vi "connection.list.vi"(8 "error in":errorcluster, 11 "Nominal Client in":refnum<class "Nominal Client.lvclass">) -> (0 "error out":errorcluster, 1 "Response":string, 2 "Nominal Connections":T1(array[cluster]), 3 "Nominal Client out":refnum<class "Nominal Client.lvclass">, 4 "Connections":T2(array[cluster]))   [LabVIEW 2024, in "nominal labview client.lvlib"]
uses:
  nominal labview client.lvlib
  <vilib>/Nominal/Nominal IO Client/Nominal Client/Nominal Client.lvclass
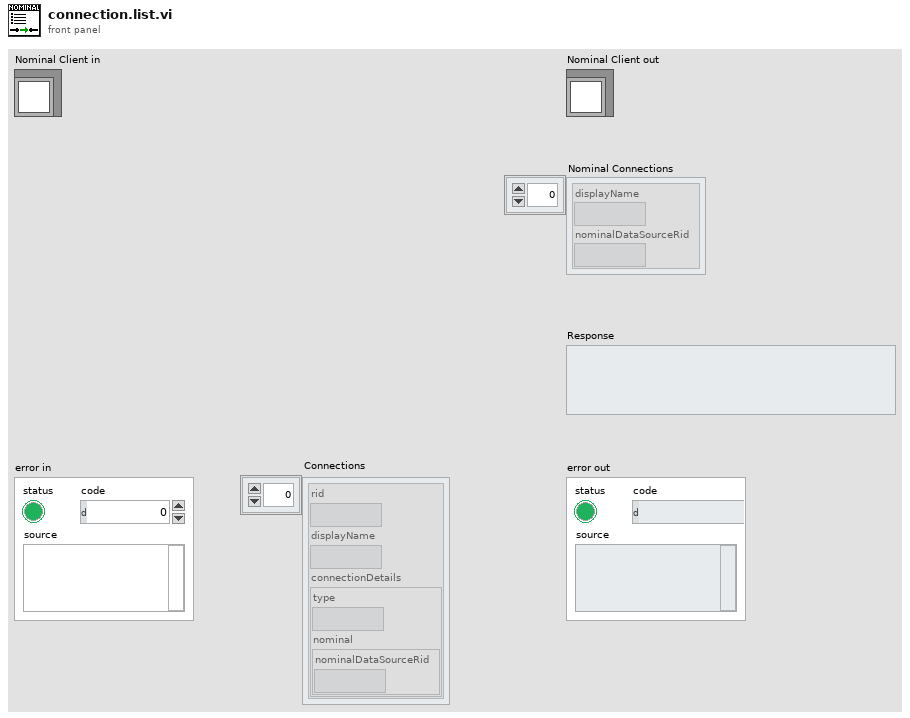
[diagram p1: front panel]
types:
  T1 = cluster{"displayName":string, "nominalDataSourceRid":string}[]
  T2 = cluster{"rid":string, "displayName":string, "connectionDetails":cluster{"type":string, "nominal":cluster{"nominalDataSourceRid":string}}}[]
  T3 = cluster{"displayName":string, "nominalDataSourceRid":string}
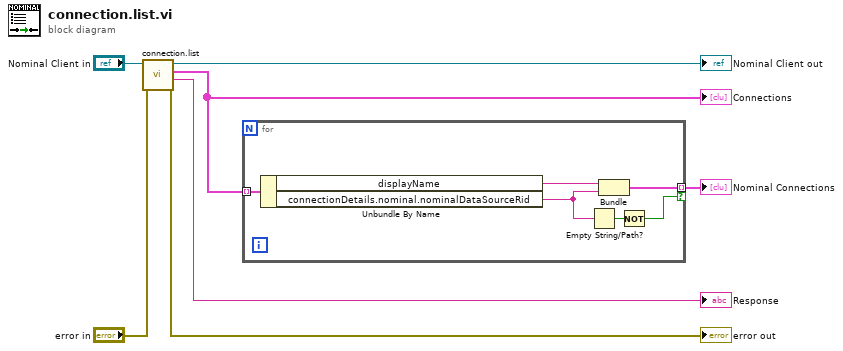
[diagram p0: block diagram]
diagram:
  n1 = call <vilib>:"connection.list.vi"("error in"="error in", "Nominal Client in"="Nominal Client in") -> ("error out"=→"error out":errorcluster, "Response"=→"Response":string, "Connections"=w2:T2, "Nominal Client out"=→"Nominal Client out":refnum<class "Nominal Client.lvclass">)  [unwired: 6 in]
  "Connections" <- w2
  n2 = for {
    tunnel: w2 -> [w13] mode=indexing
    tunnel: [w9] -> w1 mode=indexing if=w8
    n3 = Unbundle By Name(w13) -> ("displayName"=w11:string, "connectionDetails.nominal.nominalDataSourceRid"=w10:string)
    n4 = Empty String/Path?(string/path=w10) -> (empty?=w12:bool)
    n5 = Bundle("displayName"=w11, "nominalDataSourceRid"=w10) -> (w9:T3)  [unwired: 1 in]
    n6 = Not(x=w12) -> (.not. x?=w8:bool)
  }
  "Nominal Connections" <- w1
